vi "Constructor.vi"(9 "Upload ID":string, 10 "Object Key":string, 11 "Bucket":refnum<class "Bucket.lvclass">) -> (3 "Multipart Upload":refnum<class "Multipart Upload.lvclass">)   [LabVIEW 2015, in "NI_AWS_S3.lvlib" / "Multipart Upload.lvclass"]
uses:
  Multipart Upload.lvclass
  Bucket/Bucket.lvclass
  Multipart Upload.lvclass/Multipart Upload.ctl
  Write Bucket.vi
  Write Object Key.vi
  Write Upload ID.vi
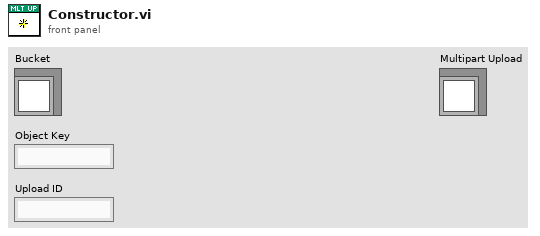
[diagram p1: front panel]
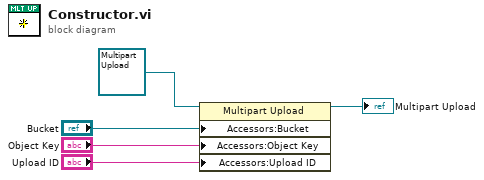
[diagram p0: block diagram]
diagram:
  n1 = property class="Multipart Upload"(reference=refnum<class "Multipart Upload.lvclass"> refnum, "Accessors:Bucket"="Bucket", "Accessors:Object Key"="Object Key", "Accessors:Upload ID"="Upload ID") -> (reference out=→"Multipart Upload":refnum<class "Multipart Upload.lvclass">)  [unwired: 1 in, 1 out]
